vi "load_LUT_from_file.vi"(2 "command_array_length":u32, 3 "input_machine_reference.lvclass":refnum<class "machine.lvclass">) -> (1 "output_machine_reference.lvclass":refnum<class "machine.lvclass">)   [LabVIEW 2014, in "machine.lvclass"]
uses:
  machine.lvclass
  machine.lvclass/machine.ctl
  dll/SCPI_LUTs.dll
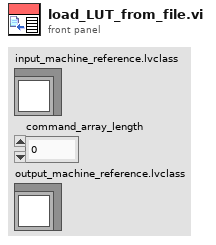
[diagram p1: front panel]
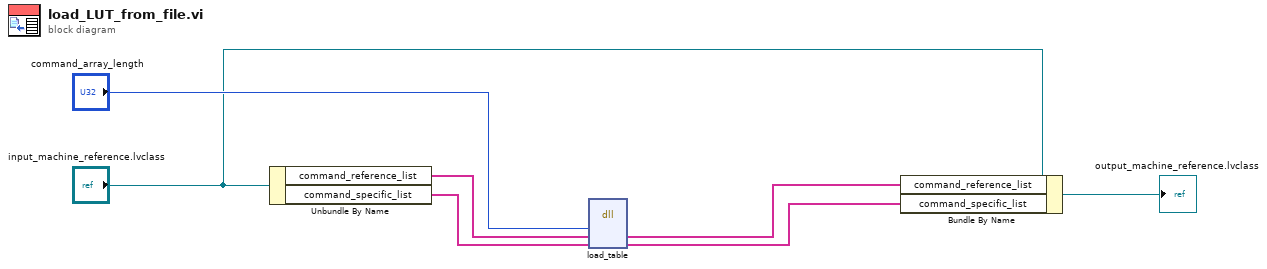
[diagram p0: block diagram]
diagram:
  n1 = Unbundle By Name("input_machine_reference.lvclass") -> ("command_reference_list"=w7:string[], "command_specific_list"=w6:string[])
  n2 = dll-call lib="C:/Users/DrippySummer/Documents/LabVIEW Data/SavaData/keithley_general_client/dll/SCPI_LUTs.dll" fn="load_table"("arr_length"="command_array_length", "SCPI_ref_arr"=w7, "SCPI_str_arr"=w6) -> ("SCPI_ref_arr"=w3:string[], "SCPI_str_arr"=w2:string[])  [unwired: 5 in, 2 out]
  n3 = Bundle By Name(cluster="input_machine_reference.lvclass", "command_reference_list"=w3, "command_specific_list"=w2) -> (→"output_machine_reference.lvclass":refnum<class "machine.lvclass">)
